vi "Sort 2D Array - Push Stack.vi"(9 "element":i32, 10 "array in":i32[](array[numeric]), 11 "top in":i32) -> (2 "array out":i32[](array[numeric]), 3 "top out":i32)   [LabVIEW 2020]
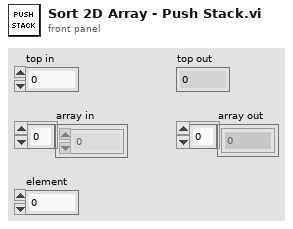
[diagram p1: front panel]
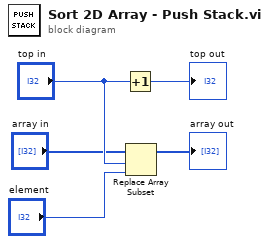
[diagram p0: block diagram]
diagram:
  n1 = Increment(x="top in") -> (x+1=→"top out":i32)
  n2 = Replace Array Subset(array="array in", new element="element", index="top in") -> (→"array out":i32[])
